vi "3_4.vi"() -> ()   [LabVIEW 2012]
panel:
  out "min index(es)":i32[](array[numeric])
  out "min value":dbl
  out "max index(es)":i32[](array[numeric])
  out "max value":dbl
  out "Результат стовбці":dbl[][](array[numeric])
  in  "Вкахіть к-сть стовпців які треба вилучити":i32
  out "Результат рядки":dbl[][](array[numeric])
  in  "Вкажіть к-сть рядків які треба вилучити":i32
  out "Значення елемента":dbl
  in  "Стовпчик":i32
  in  "Рядок":i32
  out "size(s)":i32[](array[numeric])
  out "1":dbl[][](array[numeric])
  in  "51-61":bool
  in  "stop":bool
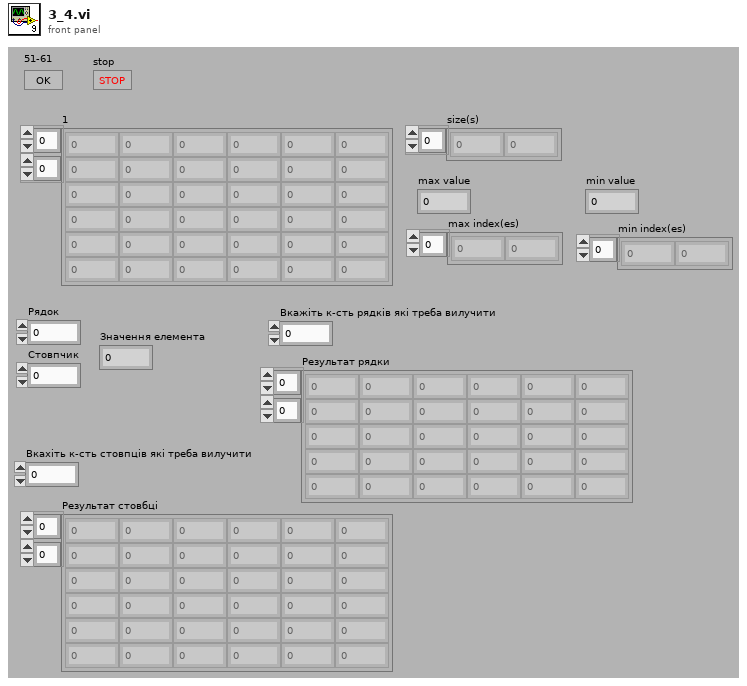
[diagram p1: front panel]
types:
  T1 = cluster{"1":dbl[][], "Size":i32[], "Результат рядки":dbl[][], "Результат стовбці":dbl[][]}
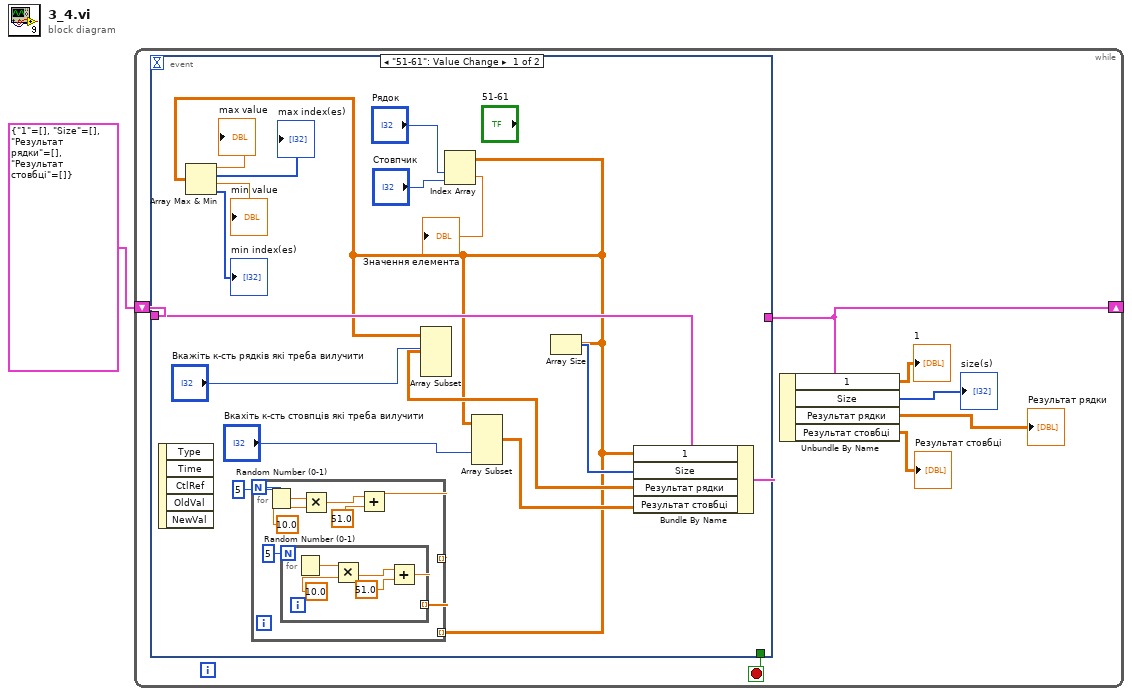
[diagram p0: block diagram]
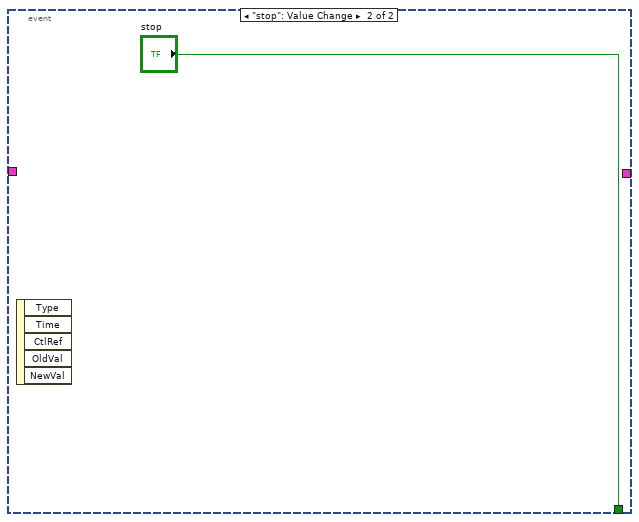
[diagram p2: hidden frame]
diagram:
  n1 = while {
    shift-right: [w6] -> _
    shift-left: T1 {"1"=[], "Size"=[], "Результат рядки"=[], "Результат стовбці"=[]} -> [w7]
    stop <- w8 stop-if-true
    n2 = event shown="[0] \"51-61\": Value Change" {
      selector: _ -> [_ _]
      dyn-events: _ -> [_ _]
      timeout: _ -> [_ _]
      tunnel: [_ "stop"] -> w8
      tunnel: w7 -> [w23 _]
      tunnel: [w22 _] -> w6
      event "51-61": Value Change {
        n3 = event-data() -> ()  [unwired: 1 in, 5 out]
        n4 = for {
          N: 5 -> [_]
          tunnel: [w25] -> _ mode=indexing
          tunnel: [w30] -> w13 mode=indexing
          n5 = Random Number (0-1)() -> (number: 0 to 1=w29:dbl)
          n6 = for {
            N: 5 -> [_]
            tunnel: [w33] -> w30 mode=indexing
            n7 = Random Number (0-1)() -> (number: 0 to 1=w34:dbl)
            n8 = Multiply(x=w34, y=10.0 ("x")) -> (x*y=w36:dbl)
            n9 = Add(x=w36, y=51.0) -> (x+y=w33:dbl)
          }
          n10 = Multiply(x=w29, y=10.0 ("x")) -> (x*y=w26:dbl)
          n11 = Add(x=w26, y=51.0) -> (x+y=w25:dbl)
        }
        n12 = Array Max & Min(array=w13) -> (max value=→"max value":dbl, max index (indices)=→"max index(es)":i32[], min value=→"min value":dbl, min index (indices)=→"min index(es)":i32[])
        n13 = Array Subset(array=w13, index (row)="Вкажіть к-сть рядків які треба вилучити") -> (w16:dbl[][])  [unwired: 3 in]
        n14 = Index Array(array=w13, index (row)="Рядок", index (col)="Стовпчик") -> (element=→"Значення елемента":dbl)
        n15 = Array Subset(array=w13, index (col)="Вкахіть к-сть стовпців які треба вилучити") -> (w14:dbl[][])  [unwired: 3 in]
        n16 = Array Size(array=w13) -> (size(s)=w21:i32[])
        n17 = Bundle By Name(cluster=w23, "1"=w13, "Size"=w21, "Результат рядки"=w16, "Результат стовбці"=w14) -> (w22:T1)
      }
      event "stop": Value Change {
        n18 = event-data() -> ()  [unwired: 1 in, 5 out]
      }
    }
    n19 = Unbundle By Name(w6) -> ("1"=→"1":dbl[][], "Size"=→"size(s)":i32[], "Результат рядки"=→"Результат рядки":dbl[][], "Результат стовбці"=→"Результат стовбці":dbl[][])
  }
